vi "Initialize Force Task.vi"(0 "NI Force Task in":refnum<class "NI Force Task.lvclass">, 1 "Force Calibration Cluster":cluster{"Left":dbl, "Right":dbl}, 2 "TDMS File":refnum<k34>, 3 "EMG info":cluster{"Collect EMG?":bool, "EMG Rate":u16}, 4 "DAQ  Channels In":T1={"Force Transducer: Left"="Dev1/ai6", "Force Transducer: Right "="Dev1/ai8", "EMG: Left"="", "EMG: Right"="", "Potentiometer: Left"="", "Potentiometer: Right"=""}, 5 "error in (no error)":errorcluster, 7 "Scanning?":bool=TRUE, 9 "Task Info In":T2={"Number of Trials"=1, "Sampling Rate (Hz)"=200, "Trial Duration (s)"=10, "Adjusted MVC (N)"=5.0, "R Phase"=0, "L Phase"=0, "L Pattern"=1, "R Pattern"=1, "Time Between Trials (s)"=5, "Lissajous Speed"=200} {"Lissajous Speed" min=1 max=200; "Time Between Trials (s)" min=1 step=1; "R Pattern" min=1 max=20 step=1; "L Pattern" min=1 max=20 step=1; "L Phase" max=360 step=1; "R Phase" max=360 step=1; "Adjusted MVC (N)" min=1.0 step=1.0; "Trial Duration (s)" min=1 step=1; "Sampling Rate (Hz)" min=1 step=1; "Number of Trials" min=1 step=1}) -> (14 "NI Force Task out":refnum<class "NI Force Task.lvclass">, 19 "error out":errorcluster)   [LabVIEW 2020, in "NI Force Task.lvlib" / "NI Force Task.lvclass"]
uses:
  NI Force Task.lvclass
  C:/Program Files/National Instruments/LabVIEW 2020/vi.lib/ActorFramework/Actor/Actor.lvclass
  Task info df.ctl
  <vilib>/ActorFramework/Message Enqueuer/Message Priority.ctl
  <vilib>/ActorFramework/Actor/Actor.lvclass/Actor.ctl
  <vilib>/ActorFramework/Message Enqueuer/Message Enqueuer.lvclass/Message Enqueuer.ctl
  NI Force Task.lvclass/NI Force Task.ctl
  NI Force Task Messages/Update Template Graph Msg/Update Template Graph Msg.lvclass/Update Template Graph Msg.ctl
  <vilib>/ActorFramework/Message Enqueuer/Init from Existing Queue.vi
  <vilib>/ActorFramework/Message Enqueuer/Enqueue.vi
  NI Force Task Messages/Update Template Graph Msg/Update Template Graph Msg.lvclass
  C:/Program Files/National Instruments/LabVIEW 2020/vi.lib/ActorFramework/Message/Message.lvclass
  <vilib>/ActorFramework/Message Priority Queue/Priority Enqueue.vi
  <vilib>/DAQmx/create/channels.llb/DAQmx Create Channel (AI-Voltage-Basic).vi
  <vilib>/DAQmx/configure/timing.llb/DAQmx Timing (Sample Clock).vi
  <vilib>/ActorFramework/Message Enqueuer/Message Enqueuer.lvclass
  <vilib>/ActorFramework/Actor/Actor.lvclass
panel:
  # "Left Arm"
  # "Right Arm"
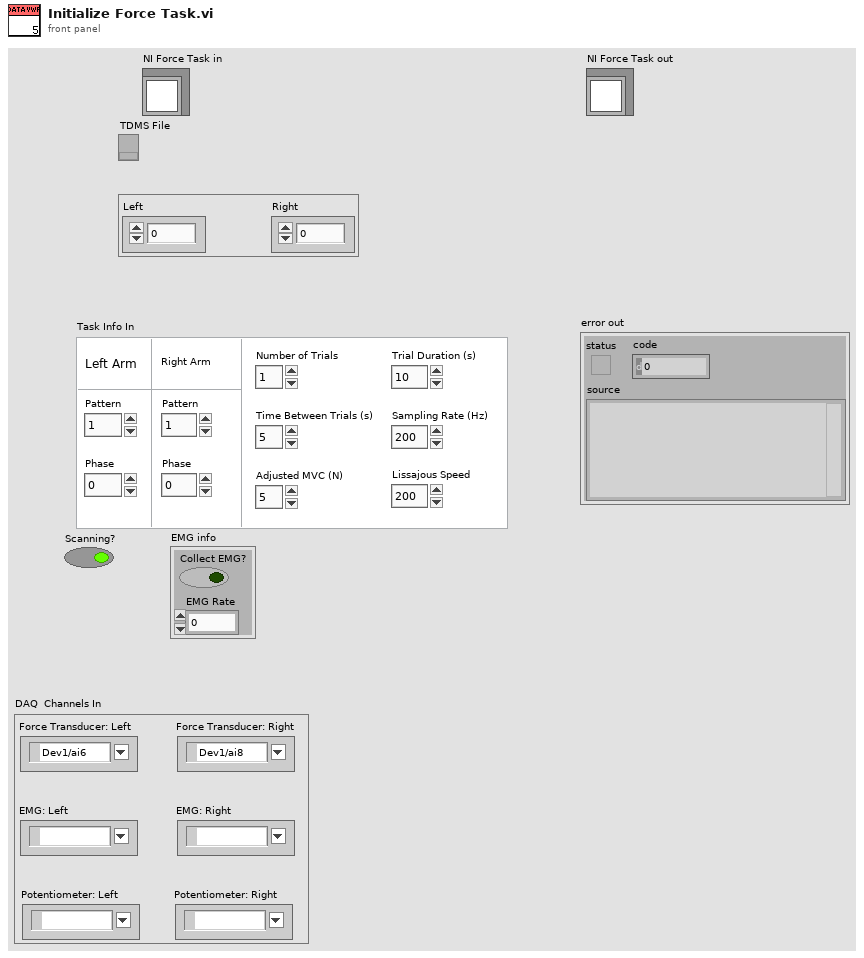
[diagram p1: front panel]
types:
  T1 = cluster{"Force Transducer: Left":tag, "Force Transducer: Right ":tag, "EMG: Left":tag, "EMG: Right":tag, "Potentiometer: Left":tag, "Potentiometer: Right":tag}
  T2 = typedef "Task info df.ctl" = cluster{"Number of Trials":u8, "Sampling Rate (Hz)":u16, "Trial Duration (s)":u8, "Adjusted MVC (N)":dbl, "R Phase":i32, "L Phase":i32, "L Pattern":u8, "R Pattern":u8, "Time Between Trials (s)":u8, "Lissajous Speed":u16}
  T3 = typedef "Actor Framework.lvlib/Message Enqueuer.lvclass/Message Priority.ctl" = enum16{"Low", "Normal", "High"}
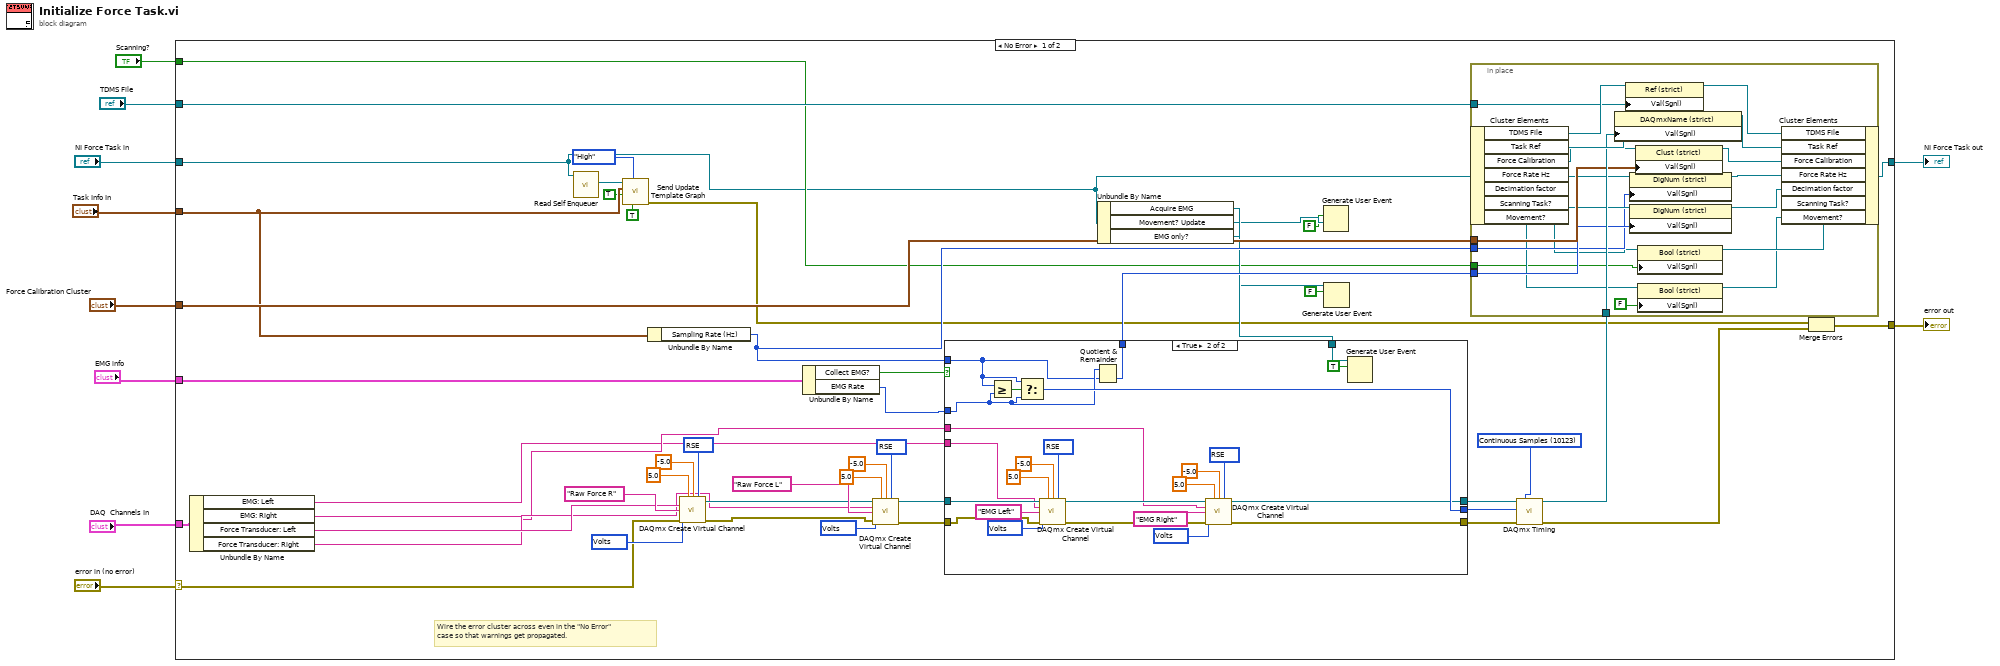
[diagram p0: block diagram]
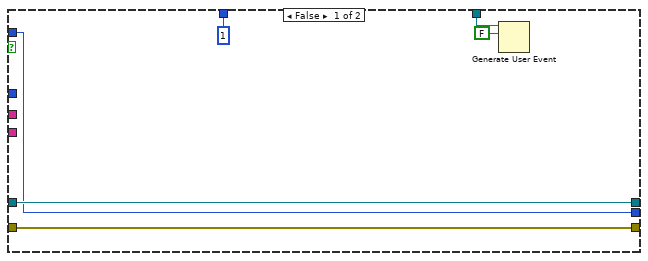
[diagram p2: hidden frame]
diagram:
  n1 = case shown="No Error" "error in (no error)" {
    selector: "error in (no error)" -> [w35 w112]
    tunnel: [w33 w112] -> w9
    tunnel: [w32 w111] -> w7
    tunnel: "NI Force Task in" -> [w15 w111]
    tunnel: "Task Info In" -> [w16 _]
    tunnel: "EMG info" -> [w58 _]
    tunnel: "DAQ  Channels In" -> [w56 _]
    tunnel: "Force Calibration Cluster" -> [w31 _]
    tunnel: "TDMS File" -> [w29 _]
    tunnel: "Scanning?" -> [w20 _]
    frame No Error {
      w36 = 10123 items=["Finite Samples"=10178, "Continuous Samples"=10123, "Hardware Timed Single Point"=12522] ("sample mode")
      w46 = 10348 items=["Volts"=10348, "From Custom Scale"=10065] ("units")
      w50 = 10083 items=["Default"=-1, "RSE"=10083, "NRSE"=10078, "Differential"=10106, "Pseudodifferential"=12529] ("input terminal configuration")
      w51 = 10348 items=["Volts"=10348, "From Custom Scale"=10065] ("units")
      w55 = 10083 items=["Default"=-1, "RSE"=10083, "NRSE"=10078, "Differential"=10106, "Pseudodifferential"=12529] ("input terminal configuration")
      # "Wire the error cluster across even in the \"No Error\"\ncase so that warnings get propagated."
      n2 = Unbundle By Name(w56) -> ("EMG: Left"=w26:tag, "EMG: Right"=w27:tag, "Force Transducer: Left"=w43:tag, "Force Transducer: Right"=w42:tag)
      n3 = call <vilib>:"Read Self Enqueuer.vi"("Actor"=w15) -> ("Self Enqueuer"=w17:refnum<class "Message Enqueuer.lvclass">)  [unwired: 10 in]
      n4 = call "Send Update Template Graph.vi"("Set Task Info?"=TRUE, "Priority"=Message_Priority."High", "Update Axes Scale"=TRUE, "Task Info In"=w16, "Message Enqueuer in"=w17) -> ("error out"=w14:errorcluster)  [unwired: 5 in, 1 out]
      n5 = Unbundle By Name(w16) -> ("Sampling Rate (Hz)"=w24:u16)
      n6 = call-poly <vilib>:"DAQmx Create Virtual Channel.vi"("maximum value"=5.0, "minimum value"=-5.0, "input terminal configuration"=w55, "physical channels"=w43, "name to assign"="Raw Force R", "units"=w51, "error in"=w35) -> ("task out"=w45:refnum<k21>, "error out"=w44:errorcluster)  [unwired: 7 in]
      n7 = Unbundle By Name(w58) -> ("Collect EMG?"=w57:bool, "EMG Rate"=w37:u16)
      n8 = call-poly <vilib>:"DAQmx Create Virtual Channel.vi"("task in"=w45, "maximum value"=5.0, "minimum value"=-5.0, "input terminal configuration"=w50, "physical channels"=w42, "name to assign"="Raw Force L", "units"=w46, "error in"=w44) -> ("task out"=w41:refnum<k21>, "error out"=w40:errorcluster)  [unwired: 6 in]
      n9 = Unbundle By Name(w15) -> ("Acquire EMG"=w23:refnum<user-event>, "Movement? Update"=w22:refnum<user-event>, "EMG only?"=w19:refnum<user-event>)
      n10 = case shown="True" w57 {
        tunnel: w41 -> [w64 w79]
        tunnel: [w64 w71] -> w39
        tunnel: [w63 w70] -> w38
        tunnel: w40 -> [w63 w78]
        tunnel: w24 -> [w62 w68]
        tunnel: w37 -> [_ w69]
        tunnel: [w62 w88] -> w28
        tunnel: w27 -> [_ w73]
        tunnel: w26 -> [_ w72]
        tunnel: [u16 1 w67] -> w25
        tunnel: w23 -> [w60 w66]
        frame False {
          n11 = Generate User Event(user event=w60, event data cluster=FALSE ("event data")) -> ()  [unwired: 2 in, 2 out]
        }
        frame True {
          w80 = 10348 items=["Volts"=10348, "From Custom Scale"=10065] ("units")
          w83 = 10083 items=["Default"=-1, "RSE"=10083, "NRSE"=10078, "Differential"=10106, "Pseudodifferential"=12529] ("input terminal configuration")
          w84 = 10348 items=["Volts"=10348, "From Custom Scale"=10065] ("units")
          w87 = 10083 items=["Default"=-1, "RSE"=10083, "NRSE"=10078, "Differential"=10106, "Pseudodifferential"=12529] ("input terminal configuration")
          n12 = Greater Or Equal?(x=w68, y=w69) -> (x >= y?=w89:bool)
          n13 = Select(t=w68, s=w89, f=w69) -> (s? t:f=w88:u16)
          n14 = call-poly <vilib>:"DAQmx Create Virtual Channel.vi"("task in"=w79, "maximum value"=5.0, "minimum value"=-5.0, "input terminal configuration"=w87, "physical channels"=w72, "name to assign"="EMG Left", "units"=w84, "error in"=w78) -> ("task out"=w77:refnum<k21>, "error out"=w76:errorcluster)  [unwired: 6 in]
          n15 = Quotient & Remainder(x=w69, y=w68) -> (floor(x/y)=w67:u16)  [unwired: 1 out]
          n16 = call-poly <vilib>:"DAQmx Create Virtual Channel.vi"("task in"=w77, "maximum value"=5.0, "minimum value"=-5.0, "input terminal configuration"=w83, "physical channels"=w73, "name to assign"="EMG Right", "units"=w80, "error in"=w76) -> ("task out"=w71:refnum<k21>, "error out"=w70:errorcluster)  [unwired: 6 in]
          n17 = Generate User Event(user event=w66, event data cluster=TRUE ("event data")) -> ()  [unwired: 2 in, 2 out]
        }
      }
      n18 = Generate User Event(user event=w22, event data cluster=FALSE ("event data")) -> ()  [unwired: 2 in, 2 out]
      n19 = Generate User Event(user event=w19, event data cluster=FALSE ("event data")) -> ()  [unwired: 2 in, 2 out]
      n20 = call-poly <vilib>:"DAQmx Timing.vi"("task/channels in"=w39, "sample mode"=w36, "rate"=w28, "error in"=w38) -> ("task out"=w30:refnum<k21>, "error out"=w34:errorcluster)  [unwired: 10 in]
      n21 = in-place {
        in-place-border: w31 -> [w102]
        in-place-border: w30 -> [w108]
        in-place-border: w29 -> [w107]
        in-place-border: w25 -> [w97]
        in-place-border: w24 -> [w96]
        in-place-border: w20 -> [w90]
        n22 = in-place-cluster #1(w15) -> ("TDMS File"=w110:refnum<vi>, "Task Ref"=w109:refnum<vi>, "Force Calibration"=w104:refnum<vi>, "Force Rate Hz"=w101:refnum<vi>, "Decimation factor"=w99:refnum<vi>, "Scanning Task?"=w95:refnum<vi>, "Movement?"=w93:refnum<vi>)
        n23 = property class="DAQmxName (strict)"(reference=w109, "Val(Sgnl)"=w108) -> (reference out=w105:refnum<vi>)  [unwired: 1 in, 1 out]
        n24 = property class="Ref (strict)"(reference=w110, "Val(Sgnl)"=w107) -> (reference out=w106:refnum<vi>)  [unwired: 1 in, 1 out]
        n25 = property class="DigNum (strict)"(reference=w101, "Val(Sgnl)"=w96) -> (reference out=w100:refnum<vi>)  [unwired: 1 in, 1 out]
        n26 = property class="DigNum (strict)"(reference=w99, "Val(Sgnl)"=w97) -> (reference out=w98:refnum<vi>)  [unwired: 1 in, 1 out]
        n27 = property class="Clust (strict)"(reference=w104, "Val(Sgnl)"=w102) -> (reference out=w103:refnum<vi>)  [unwired: 1 in, 1 out]
        n28 = property class="Bool (strict)"(reference=w95, "Val(Sgnl)"=w90) -> (reference out=w94:refnum<vi>)  [unwired: 1 in, 1 out]
        n29 = property class="Bool (strict)"(reference=w93, "Val(Sgnl)"=FALSE ("Value (Signaling)")) -> (reference out=w92:refnum<vi>)  [unwired: 1 in, 1 out]
        n30 = in-place-cluster #1("TDMS File"=w106, "Task Ref"=w105, "Force Calibration"=w103, "Force Rate Hz"=w100, "Decimation factor"=w98, "Scanning Task?"=w94, "Movement?"=w92) -> (w32:refnum<class "NI Force Task.lvclass">)
      }
      n31 = Merge Errors(w14, w34) -> (w33:errorcluster)
    }
    frame Error {
    }
  }
  "error out" <- w9
  "NI Force Task out" <- w7
